vi "Initialize KH Array.vi"(10 "KH #":u16[](array[numeric]), 11 "Control in":variant) -> (3 "Control out":variant)   [LabVIEW 2016, in "Control Experiment.lvclass"]
uses:
  Control Experiment.lvclass
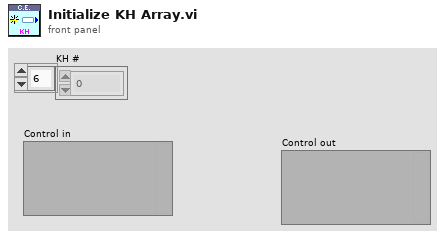
[diagram p1: front panel]
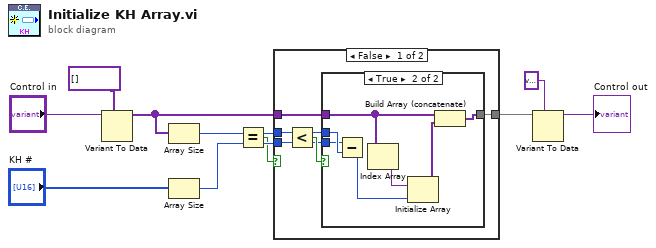
[diagram p0: block diagram]
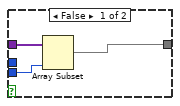
[diagram p2: hidden frame]
diagram:
  n1 = Variant To Data(type=variant[] [], Variant="Control in") -> (data=w4:variant[])  [unwired: 1 in, 1 out]
  n2 = Array Size(array=w4) -> (size(s)=w10:i32)
  n3 = Array Size(array="KH #") -> (size(s)=w9:i32)
  n4 = Equal?(x=w10, y=w9) -> (x = y?=w7:bool)
  n5 = case shown="False" w7 {
    tunnel: [w11 w26] -> w2
    tunnel: w4 -> [w12 w26]
    tunnel: w9 -> [w13 _]
    tunnel: w10 -> [w14 _]
    frame False {
      n6 = Less?(x=w14, y=w13) -> (x < y?=w15:bool)
      n7 = case shown="True" w15 {
        tunnel: w14 -> [_ w20]
        tunnel: w13 -> [w17 w19]
        tunnel: w12 -> [w18 w24]
        tunnel: [w16 w23] -> w11
        frame False {
          n8 = Array Subset(array=w18, length=w17) -> (w16:variant[])  [unwired: 1 in]
        }
        frame True {
          n9 = Subtract(x=w19, y=w20) -> (x-y=w25:i32)
          n10 = Index Array(array=w24) -> (element=w21:variant)  [unwired: 1 in]
          n11 = Initialize Array(w21, w25) -> (w22:variant[])
          n12 = Build Array (concatenate)(w24, w22) -> (w23:variant[])
        }
      }
    }
    frame True {
    }
  }
  n13 = Variant To Data(type=variant, Variant=w2) -> (data=→"Control out":variant)  [unwired: 1 in, 1 out]
